vi "downsample 1D array - double.vi"(2 "Ave N":dbl, 3 "Array In":dbl[](array[numeric])) -> (1 "Array Out":dbl[](array[numeric]))   [LabVIEW 2014]
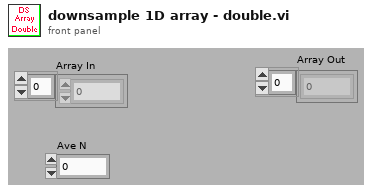
[diagram p1: front panel]
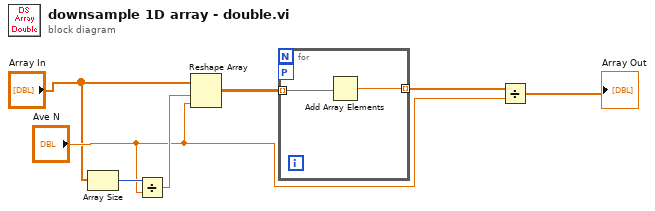
[diagram p0: block diagram]
diagram:
  n1 = Array Size(array="Array In") -> (size(s)=w7:i32)
  n2 = Divide(x=w7, y="Ave N") -> (x/y=w5:dbl)
  n3 = Reshape Array("Array In", w5, "Ave N") -> (w4:dbl[][])
  n4 = for {
    tunnel: w4 -> [w9] mode=indexing
    tunnel: [w8] -> w6 mode=indexing
    workers-P: _ -> [_]
    n5 = Add Array Elements(numeric array=w9) -> (sum=w8:dbl)
  }
  n6 = Divide(x=w6, y="Ave N") -> (x/y=→"Array Out":dbl[])
